vi "Read heartbeat.vi"(8 "error in (no error)":errorcluster, 11 "TCSPublicStatus in":refnum<class "TCSTcsStatus.lvclass">) -> (0 "error out":errorcluster, 2 "heartbeat":u32, 3 "TCSPublicStatus out":refnum<class "TCSTcsStatus.lvclass">)   [LabVIEW 2022 SP3, in "TCSDataDefinitions.lvlib" / "TCSPublicStatus.lvlib" / "TCSTcsStatus.lvclass"]
uses:
  TCSTcsStatus.lvclass
  TCSTcsStatus.lvclass/TCSTcsStatus.ctl
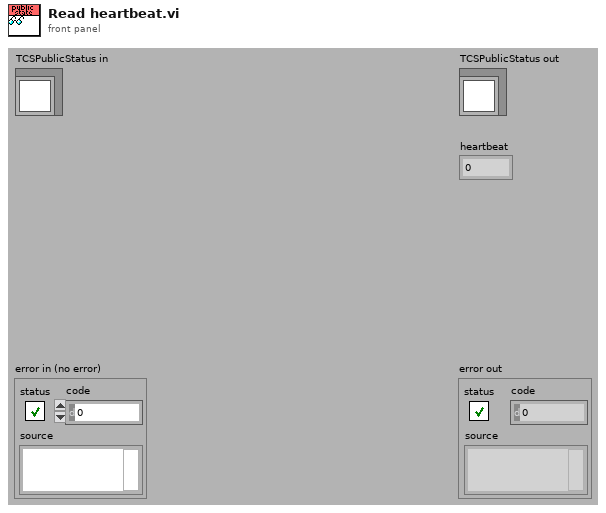
[diagram p1: front panel]
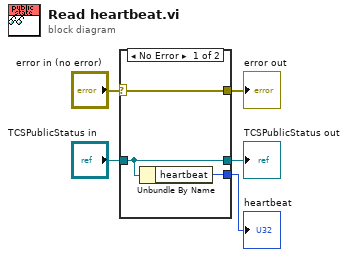
[diagram p0: block diagram]
diagram:
  n1 = case shown="No Error" "error in (no error)" {
    selector: "error in (no error)" -> [w8 w9]
    tunnel: [w8 w9] -> w4
    tunnel: [w7 w10] -> w2
    tunnel: "TCSPublicStatus in" -> [w7 w10]
    tunnel: [w6 _] -> w1
    frame No Error {
      n2 = Unbundle By Name(w7) -> ("heartbeat"=w6:u32)
    }
    frame Error {
    }
  }
  "error out" <- w4
  "TCSPublicStatus out" <- w2
  "heartbeat" <- w1
